vi "writeToBinary.vi"(0 "cropLinesOut":dbl=1.0, 1 "File control":T3={"Subject ID"="test", "Eye"=FALSE, "Output Path"=path "E:/test", "String"="OS", "String 2"="OD"}, 5 "Scan":refnum<class "Scan.lvclass">, 7 "Memory (GB)":dbl format="%#_3g", 9 "Updated camera":T2, 11 "error in":errorcluster, 12 "Progress":refnum<vi>) -> (4 "Output Path":path, 6 "OCT filename out":string, 10 "Camera out":T2, 15 "error out":errorcluster)   [LabVIEW 2017]
uses:
  <vilib>/vision/Image Controls.llb/IMAQ Image.ctl
  classes/Scans/Scan.lvclass
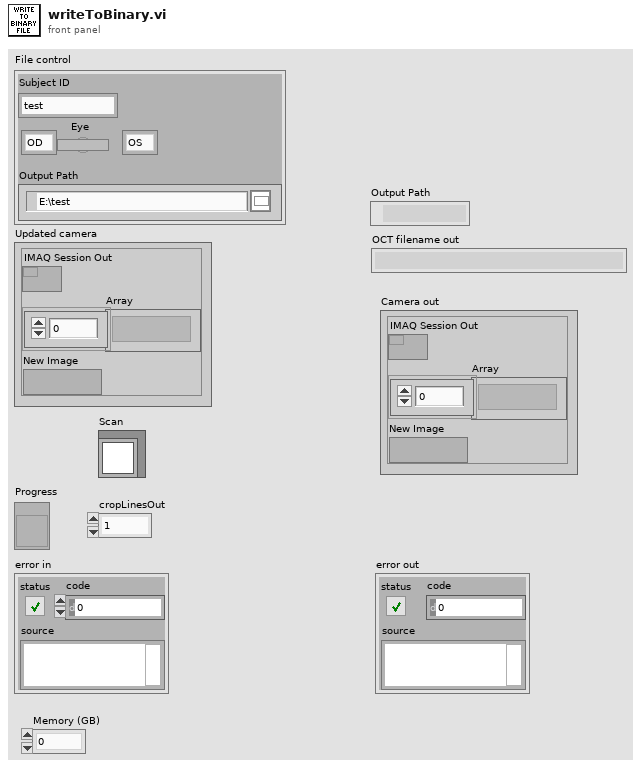
[diagram p1: front panel]
types:
  T1 = typedef "IMAQ Image.ctl" = refnum<image>
  T2 = cluster{"IMAQ Session Out":refnum<k11>, "Array":T1[], "New Image":T1}
  T3 = cluster{"Subject ID":string, "Eye":bool, "Output Path":path, "String":string, "String 2":string}
  T4 = enum16{"big-endian, network order", "native, host order", "little-endian"}
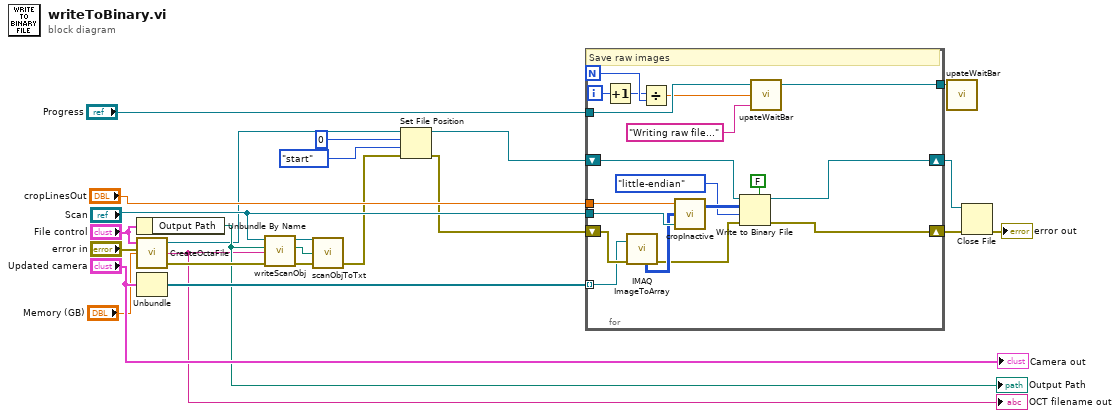
[diagram p0: block diagram]
diagram:
  n1 = Unbundle By Name("File control") -> ("Output Path"=w11:path)
  "Output Path" <- w11
  n2 = call "CreateOctaFile.vi"("error in"="error in", "Memory (GB)"="Memory (GB)", "File control"="File control") -> ("error out"=w21:errorcluster, "OCT filename out"=w10:string, "OCTA refnum out"=w6:refnum<file>)
  "OCT filename out" <- w10
  n3 = Unbundle("Updated camera") -> ("Array"=w23:T1[])  [unwired: 2 out]
  n4 = call "writeScanObj.vi"("error in"=w21, "OCT filename in"=w10, "Output Path"=w11, "Scan"="Scan") -> ("error out"=w14:errorcluster, "ScanObj ffname"=w13:path, "Scan out"=w12:refnum<class "Scan.lvclass">)  [unwired: 1 in]
  n5 = call "scanObjToTxt.vi"("error in (no error)"=w14, "Path"=w13, "Scan"=w12) -> ("error out"=w5:errorcluster)  [unwired: 2 in]
  n6 = Set File Position(offset (in bytes) (0)=i64 0, refnum=w6, from (0:start)=enum16{"start", "end", "current"}."start", error in=w5) -> (refnum out=w2:refnum<file>, error out=w1:errorcluster)
  n7 = for {
    N -> [w43]
    tunnel: w23 -> [w27] mode=indexing
    shift-right: [w28] -> w17
    shift-left: w1 -> [w42]
    tunnel: "Scan" -> [w39]
    tunnel: "Progress" -> [w33]
    tunnel: [w30] -> w16
    tunnel: "cropLinesOut" -> [w26]
    shift-right: [w25] -> w18
    shift-left: w2 -> [w34]
    i -> [w40]
    # "Save raw images"
    n8 = Increment(x=w40) -> (x+1=w41:i32)
    n9 = call "IMAQ ImageToArray"("error in (no error)"=w42, "Image"=w27) -> ("Image Pixels (U16)"=w38:u16[][], "error out"=w36:errorcluster)  [unwired: 2 in, 3 out]
    n10 = Divide(x=w41, y=w43) -> (x/y=w32:dbl)
    n11 = call "cropInactive.vi"("Scan in"=w39, "Whole camera frame"=w38, "cropLines"=w26) -> ("Cropped camera frame"=w37:u16[][])  [unwired: 1 in]
    n12 = Write to Binary File(file (use dialog)=w34, data=w37, error in=w36, 5:FALSE ("prepend array or string size? (T)"), 9:T4."little-endian" ("byte order (0:big-endian, network order)")) -> (refnum out=w25:refnum<file>, error out=w28:errorcluster)  [unwired: 1 in, 1 out]
    n13 = call "upateWaitBar.vi"("waitbar text"="Writing raw file...", "waitbar value [0,1]"=w32, "Progress"=w33) -> ("Updated Progress"=w30:refnum<vi>)  [unwired: 2 in]
  }
  n14 = call "upateWaitBar.vi"("Progress"=w16) -> ()  [unwired: 4 in, 1 out]
  n15 = Close File(refnum=w18, error in=w17) -> (error out=→"error out":errorcluster)  [unwired: 1 out]
  "Camera out" <- "Updated camera"
